vi "utility_get_rt_modules_and_channels.vi"(11 "IP Adress":string="localhost" caption="IP地址") -> (1 "Device Tree Items":T1(array[cluster]) caption="设备树项目")   [LabVIEW 2015]
uses:
  <resource>/objmgr/ni.var.rc
  <resource>/objmgr/cRIO.rc
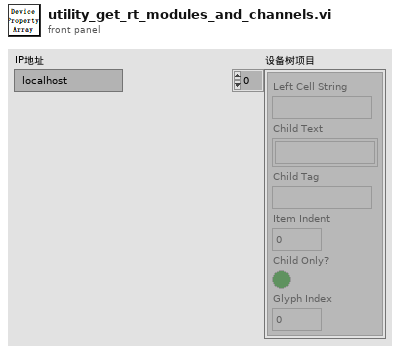
[diagram p1: front panel]
types:
  T1 = cluster{"Left Cell String":string, "Child Text":string[], "Child Tag":string, "Item Indent":i32, "Child Only?":bool, "Glyph Index":i32}[]
  T2 = cluster{"Left Cell String":string, "Child Text":string[], "Child Tag":string, "Item Indent":i32, "Child Only?":bool, "Glyph Index":i32}
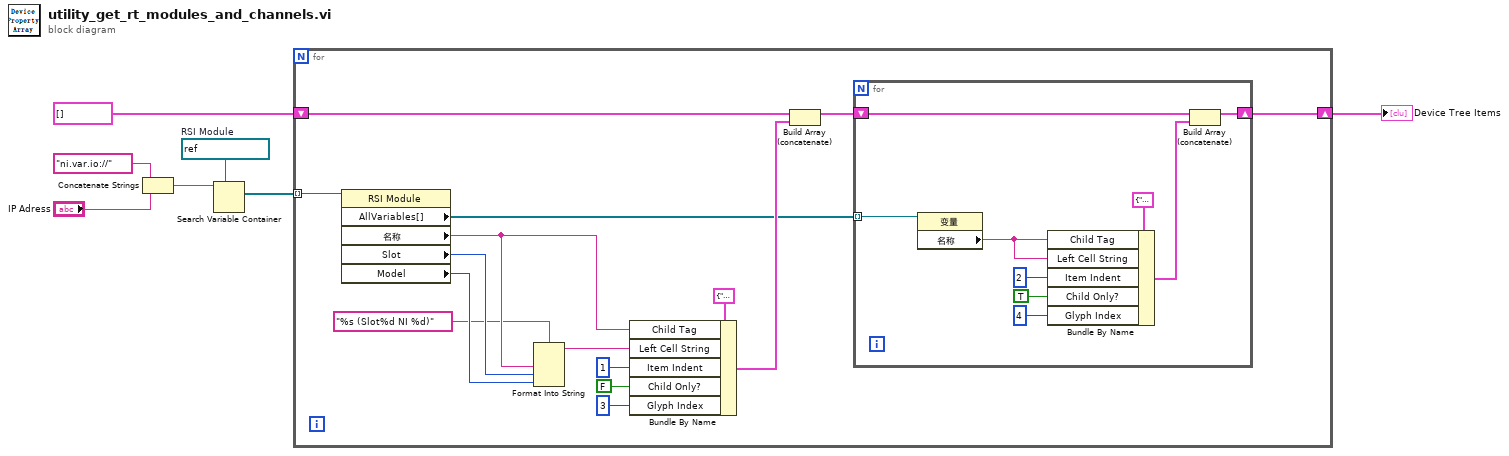
[diagram p0: block diagram]
diagram:
  w7 = refnum<k21> refnum  # RSI Module
  n1 = Concatenate Strings("ni.var.io://", "IP Adress") -> (w5:string)
  n2 = Search Variable Container(7:w7, 11:w5) -> (2:w4:refnum<k21>[])  [unwired: 4 in, 2 out]
  n3 = for {
    tunnel: w4 -> [w22] mode=indexing
    shift-right: [w18] -> w1
    shift-left: T1 [] ("多项") -> [w20]
    n4 = property class="RSI Module"(reference=w22) -> ("AllVariables[]"=w17:refnum<k21>[], "名称"=w14:string, "Slot"=w16:u32, "Model"=w15:u32)  [unwired: 1 in, 2 out]
    n5 = Format Into String(format string="%s (Slot%d NI %d)" ("格式字符串"), w14, w16, w15) -> (resulting string=w13:string)  [unwired: 2 in, 1 out]
    n6 = Bundle By Name(cluster=T2 {"Left Cell String"="", "Child Text"=[], "Child Tag"="", "Item Indent"=0, "Child Only?"=FALSE, "Glyph Index"=0} ("Item"), "Child Tag"=w14, "Left Cell String"=w13, "Item Indent"=1, "Child Only?"=FALSE, "Glyph Index"=3) -> (w21:T2)
    n7 = Build Array (concatenate)(w20, w21) -> (w19:T1)
    n8 = for {
      tunnel: w17 -> [w31] mode=indexing
      shift-right: [w28] -> w18
      shift-left: w19 -> [w29]
      n9 = property class="变量"(reference=w31) -> ("名称"=w23:string)  [unwired: 1 in, 2 out]
      n10 = Bundle By Name(cluster=T2 {"Left Cell String"="", "Child Text"=[], "Child Tag"="", "Item Indent"=0, "Child Only?"=FALSE, "Glyph Index"=0} ("Item"), "Child Tag"=w23, "Left Cell String"=w23, "Item Indent"=2, "Child Only?"=TRUE, "Glyph Index"=4) -> (w30:T2)
      n11 = Build Array (concatenate)(w29, w30) -> (w28:T1)
    }
  }
  "Device Tree Items" <- w1
